vi "ProducerConsumer_SendDataToProducer.vi"() -> ()   [LabVIEW 2015]
doc: "Use this template to build a producer/consumer design pattern with events to produce queue items. Use this design pattern instead of the User Interface Event Handler pattern for user interfaces when you want to execute code asynchronously in response to an event without slowing the user interface responsiveness."
panel:
  out "element out 2":string
  out "element out":string
  in  "element in":string="element"
  in  "Queue Event":bool
  in  "stop":bool
  # "Producer Send \nData to Consumer"
  # "Producer Receive\nData from Consumer"
  # "Consumer Receive\nData from Producer"
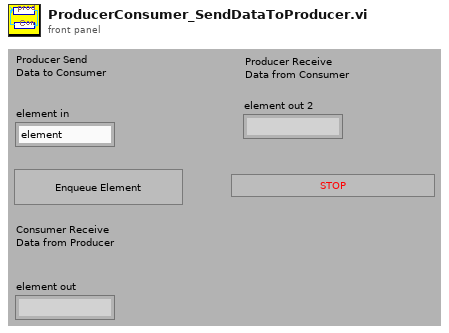
[diagram p1: front panel]
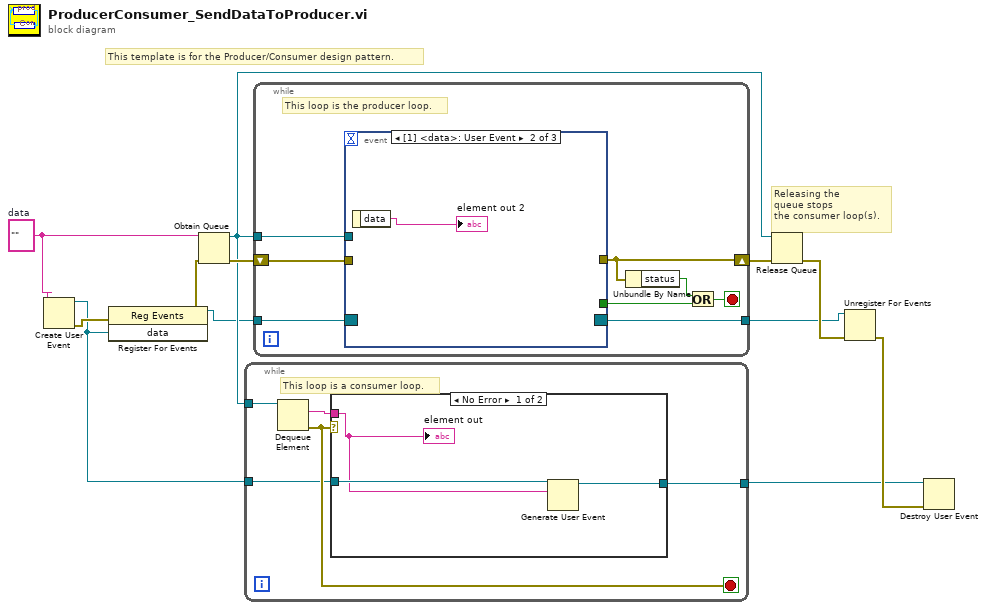
[diagram p0: block diagram]
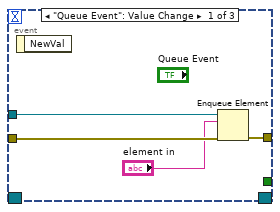
[diagram p3: hidden frame]
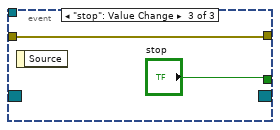
[diagram p4: hidden frame]
diagram:
  w9 = ""  # data
  # "Releasing the\nqueue stops\nthe consumer loop(s)."
  # "This template is for the Producer/Consumer design pattern."
  n1 = Create User Event(user event datatype=w9) -> (user event=w5:refnum<user-event>, error out=w7:errorcluster)  [unwired: 1 in]
  n2 = register-events(error in=w7, w5) -> (reference out=w6:refnum<event-registration>, error out=w8:errorcluster)  [unwired: 1 in]
  n3 = Obtain Queue(element data type=w9, error in (no error)=w8) -> (queue out=w10:refnum<queue>, error out=w12:errorcluster)  [unwired: 2 in, 2 out]
  n4 = while {
    tunnel: w10 -> [w17]
    tunnel: w5 -> [w14]
    tunnel: [w13] -> w1
    stop <- w16 stop-if-true
    # "This loop is a consumer loop."
    n5 = Dequeue Element(queue=w17) -> (element=w15:string, error out=w16:errorcluster)  [unwired: 1 in, 3 out]
    n6 = case shown="No Error" w16 {
      tunnel: w15 -> [w18 _]
      tunnel: w14 -> [w20 w21]
      tunnel: [w19 w21] -> w13
      frame No Error {
        n7 = Generate User Event(user event=w20, event data cluster=w18) -> (user event out=w19:refnum<user-event>)  [unwired: 2 in, 1 out]
        "element out" <- w18
      }
      frame Error {
      }
    }
  }
  n8 = while {
    shift-right: [w25] -> w11
    shift-left: w12 -> [w28]
    tunnel: w10 -> [w29]
    tunnel: w6 -> [w23]
    tunnel: [w22] -> w3
    stop <- w26 stop-if-true
    # "This loop is the producer loop."
    n9 = event shown="[1] <data>: User Event" {
      selector: w23 -> [_ _ _]
      dyn-events: [_ _ _] -> w22
      timeout: _ -> [_ _ _]
      tunnel: w29 -> [w33 _ _]
      tunnel: w28 -> [w32 _ w35]
      tunnel: [w31 _ w35] -> w25
      tunnel: [_ _ "stop"] -> w27
      event "Queue Event": Value Change {
        n10 = event-data() -> ()  [unwired: 2 out]
        n11 = Enqueue Element(queue=w33, element="element in", error in (no error)=w32) -> (error out=w31:errorcluster)  [unwired: 3 out]
      }
      event User Event {
        n12 = event-data() -> ("data"=→"element out 2":string)  [unwired: 1 out]
      }
      event "stop": Value Change {
        n13 = event-data() -> ()  [unwired: 2 out]
      }
    }
    n14 = Unbundle By Name(w25) -> ("status"=w24:bool)
    n15 = Or(x=w24, y=w27) -> (x .or. y?=w26:bool)
  }
  n16 = Release Queue(queue=w10, error in (no error)=w11) -> (error out=w4:errorcluster)  [unwired: 3 out]
  n17 = Unregister For Events(event registration refnum=w3, error in=w4) -> (error out=w2:errorcluster)
  n18 = Destroy User Event(user event=w1, error in=w2) -> ()  [unwired: 1 out]
